vi "_TreeItem.Property.Get.Dictionary.Read.vi"(8 "error in (no error)":errorcluster, 9 "Keys":string[](array[string]), 10 "Type":string, 11 "DictionaryProperty":refnum<k39>) -> (0 "error out":errorcluster, 2 "Dictionary Variant":variant, 3 "DictionaryProperty out":refnum<k39>)   [LabVIEW 2027, in "Advanced System Definition.lvlib"]
uses:
  SysDef API/Advanced System Definition.lvlib
  C:/NetCoreDLL/NationalInstruments.VeriStand.SystemStorage.dll
  NetCoreDLL/NationalInstruments.VeriStand.SystemStorage.dll
  _Types/Dictionary Item.ctl
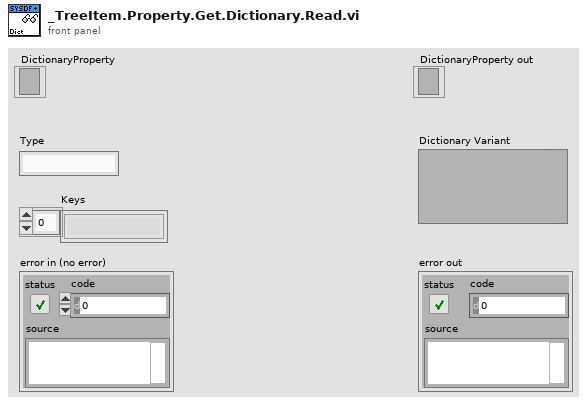
[diagram p1: front panel]
types:
  T1 = typedef "Advanced System Definition.lvlib/Dictionary Item.ctl" = cluster{"index":i32, "key":string, "value":variant}
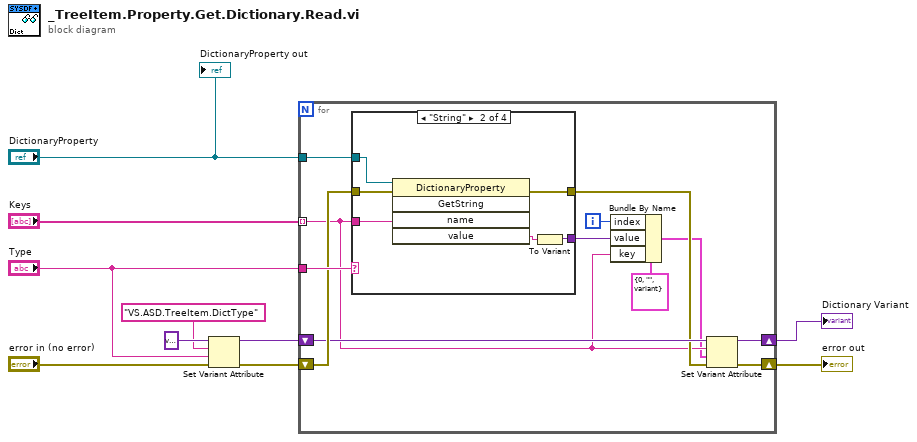
[diagram p0: block diagram]
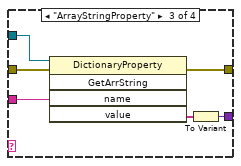
[diagram p3: hidden frame]
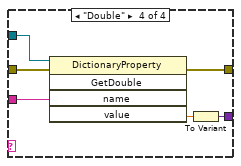
[diagram p4: hidden frame]
diagram:
  n1 = Set Variant Attribute(Variant=variant, name="VS.ASD.TreeItem.DictType", value="Type", error in="error in (no error)") -> (Variant out=w1:variant, error out=w2:errorcluster)  [unwired: 1 out]
  n2 = for {
    tunnel: "Type" -> [w22]
    tunnel: "DictionaryProperty" -> [w21]
    tunnel: "Keys" -> [w14] mode=indexing
    shift-right: [w16] -> w9
    shift-left: w2 -> [w20]
    shift-right: [w18] -> w7
    shift-left: w1 -> [w19]
    i -> [w13]
    n3 = case shown="\"String\"" w22 {
      tunnel: w21 -> [_ w29 w35 w41]
      tunnel: w20 -> [w23 w28 w34 w40]
      tunnel: [w23 w27 w32 w39] -> w17
      tunnel: w14 -> [_ w26 w31 w38]
      tunnel: [_ w24 w30 w36] -> w12
      frame Default {
      }
      frame "String" {
        n4 = invoke class="DictionaryProperty" method="GetString"(reference=w29, error in=w28, "name"=w26) -> (error out=w27:errorcluster, "value"=w25:string)  [unwired: 2 in, 3 out]
        n5 = To Variant(anything=w25) -> (Variant=w24:variant)
      }
      frame "ArrayStringProperty" {
        n6 = invoke class="DictionaryProperty" method="GetArrString"(reference=w35, error in=w34, "name"=w31) -> (error out=w32:errorcluster, "value"=w33:string[])  [unwired: 2 in, 3 out]
        n7 = To Variant(anything=w33) -> (Variant=w30:variant)
      }
      frame "Double" {
        n8 = invoke class="DictionaryProperty" method="GetDouble"(reference=w41, error in=w40, "name"=w38) -> (error out=w39:errorcluster, "value"=w37:dbl)  [unwired: 2 in, 3 out]
        n9 = To Variant(anything=w37) -> (Variant=w36:variant)
      }
    }
    n10 = Bundle By Name(cluster=T1 {"index"=0, "key"="", "value"=variant(string "")} ("Dictionary String Item"), "index"=w13, "value"=w12, "key"=w14) -> (w11:T1)
    n11 = Set Variant Attribute(Variant=w19, name=w14, value=w11, error in=w17) -> (Variant out=w18:variant, error out=w16:errorcluster)  [unwired: 1 out]
  }
  "Dictionary Variant" <- w7
  "error out" <- w9
  "DictionaryProperty out" <- "DictionaryProperty"
